vi "onDisconnection.vi"(8 "error in (no error)":errorcluster, 11 "Connection.LocalQueue":refnum<class "Connection.NetworkStream.lvclass">) -> (0 "error out":errorcluster, 3 "No Connection":refnum<class "Connection.NetworkStream.lvclass">)   [LabVIEW 2013, in "Connection.NetworkQueue_GOSPL.lvlib" / "Connection.NetworkStream.lvclass"]
uses:
  Connection.NetworkStream/Connection.NetworkStream.lvclass
  Connection/Connection.lvclass
  Connection.NetworkStream/Connection.NetworkStream.lvclass/Connection.NetworkStream.ctl
  <resource>/objmgr/ni.dex.rc
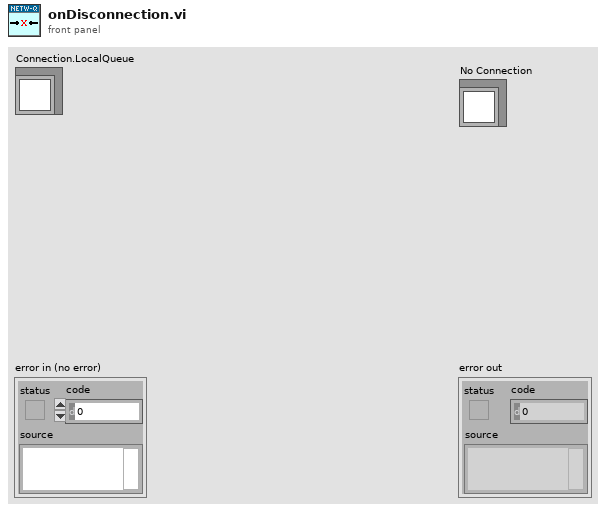
[diagram p1: front panel]
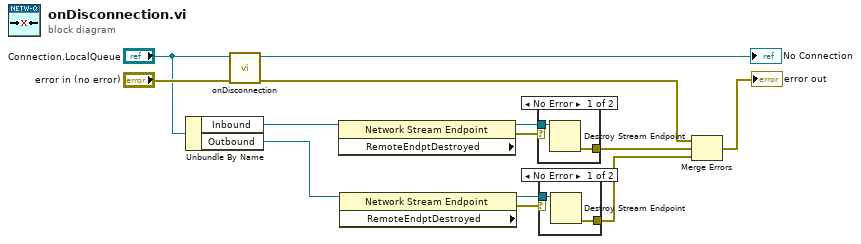
[diagram p0: block diagram]
diagram:
  n1 = Unbundle By Name("Connection.LocalQueue") -> ("Inbound"=w7:refnum<k21>, "Outbound"=w2:refnum<k21>)
  n2 = call-parent "onDisconnection.vi"("error in (no error)"="error in (no error)", "Connection"="Connection.LocalQueue") -> ("error out"=w11:errorcluster, "No connection"=→"No Connection":refnum<class "Connection.NetworkStream.lvclass">)  [unwired: 8 in]
  n3 = property class="Network Stream Endpoint" props=["RemoteEndptDestroyed"](reference=w7) -> (reference out=w6:refnum<k21>, error out=w5:errorcluster)  [unwired: 1 in, 1 out]
  n4 = property class="Network Stream Endpoint" props=["RemoteEndptDestroyed"](reference=w2) -> (reference out=w3:refnum<k21>, error out=w4:errorcluster)  [unwired: 1 in, 1 out]
  n5 = case shown="No Error" w5 {
    tunnel: [w15 _] -> w8
    tunnel: w6 -> [w14 _]
    frame No Error {
      n6 = Destroy Stream Endpoint(11:w14) -> (0:w15:errorcluster)  [unwired: 1 in]
    }
    frame Error {
    }
  }
  n7 = case shown="No Error" w4 {
    tunnel: [w17 _] -> w1
    tunnel: w3 -> [w16 _]
    frame No Error {
      n8 = Destroy Stream Endpoint(11:w16) -> (0:w17:errorcluster)  [unwired: 1 in]
    }
    frame Error {
    }
  }
  n9 = Merge Errors(w11, w8, w1) -> (→"error out":errorcluster)
